vi "ABOUT SCREEN Unitest.vi"(8 "error in (no error)":errorcluster) -> (0 "error out":errorcluster)   [LabVIEW 2025]
panel:
  out "version":string="v1.AU.26"
  out "reference out":refnum<vi>
  in  "close":bool
  in  "Tab Selection":enum32{"About", "License", "Company"}(radio) caption="Radio Buttons - Customizable"
  out "Tab Control":T1(tab)
  out "Operating System":string="Windows 11 Pro"
  out "Version":string="1.AU.26"
  out "Workorder":string="2479"
  out "Runtime":string="LabVIEW 2025 (64-bit)"
  out "Instrument Serial":string="770073"
  out "Firmware Version":string="BCLV 3.6"
  # "v"
  # "© Copyright 2023 | Paltro Inc."
  # "All rights reserved."
  # "Version"
  # "Workorder"
  # "Runtime"
  # "Copyright"
  # "© 2023"
  # "Firmware Version"
  # "Operating System"
  # "Instrument Serial"
  # "Status"
  # "."
  # "Active"
  # "Licence Type"
  # "Single-seat commercial"
  # "Seats"
  # "1 of 1 in use"
  # "Expires"
  # "Perpetual"
  # "MANUFACTURER"
  # "Company"
  # "hello@palto.com"
  # "Mail"
  # "www.paltro.com"
  # "Website"
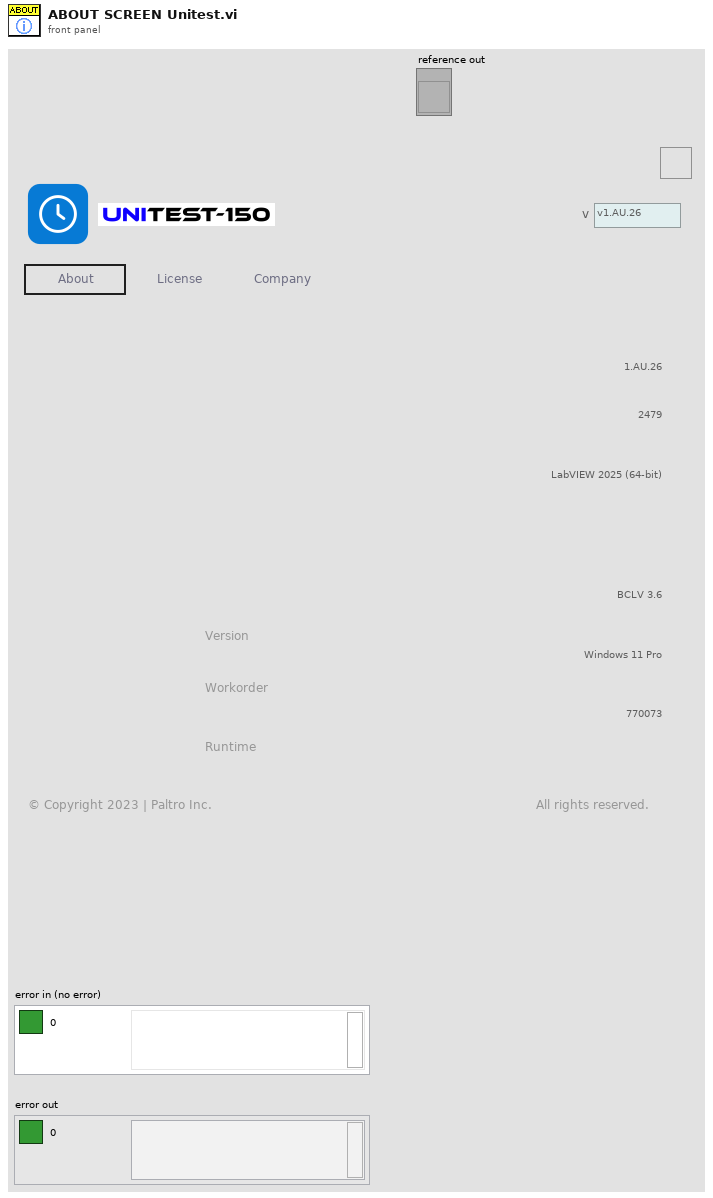
[diagram p1: front panel]
types:
  T1 = enum32{"About", "License", "Company", "System info"}
  T2 = enum32{"Invalid", "Standard", "Closed", "Hidden", "Minimized", "Maximized"}
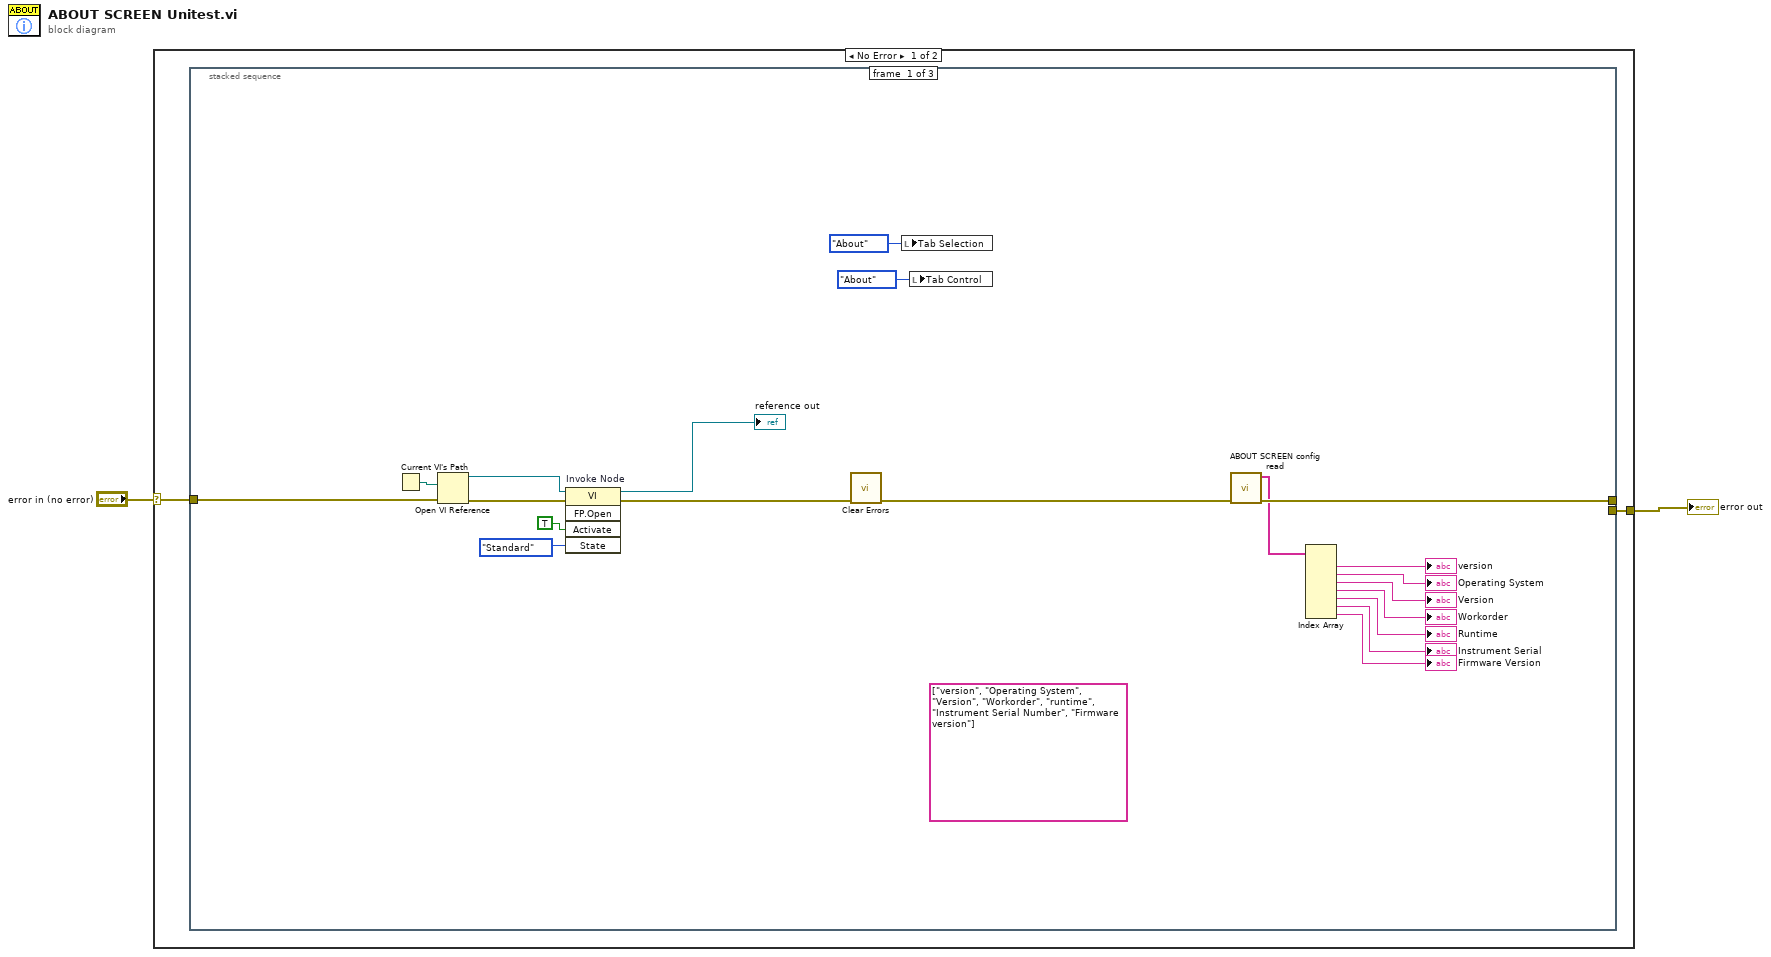
[diagram p0: block diagram]
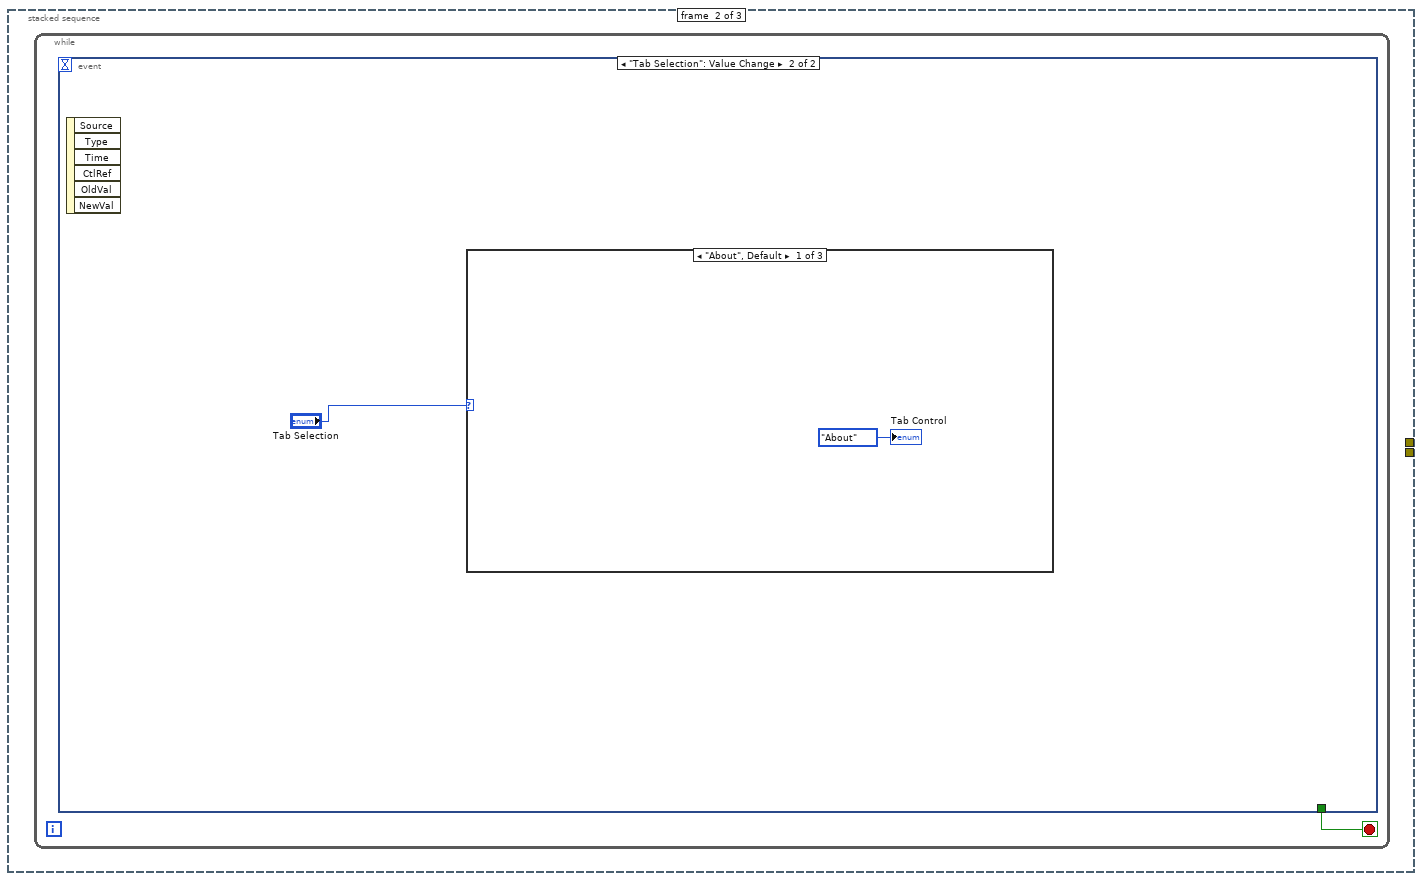
[diagram p2: hidden frame]
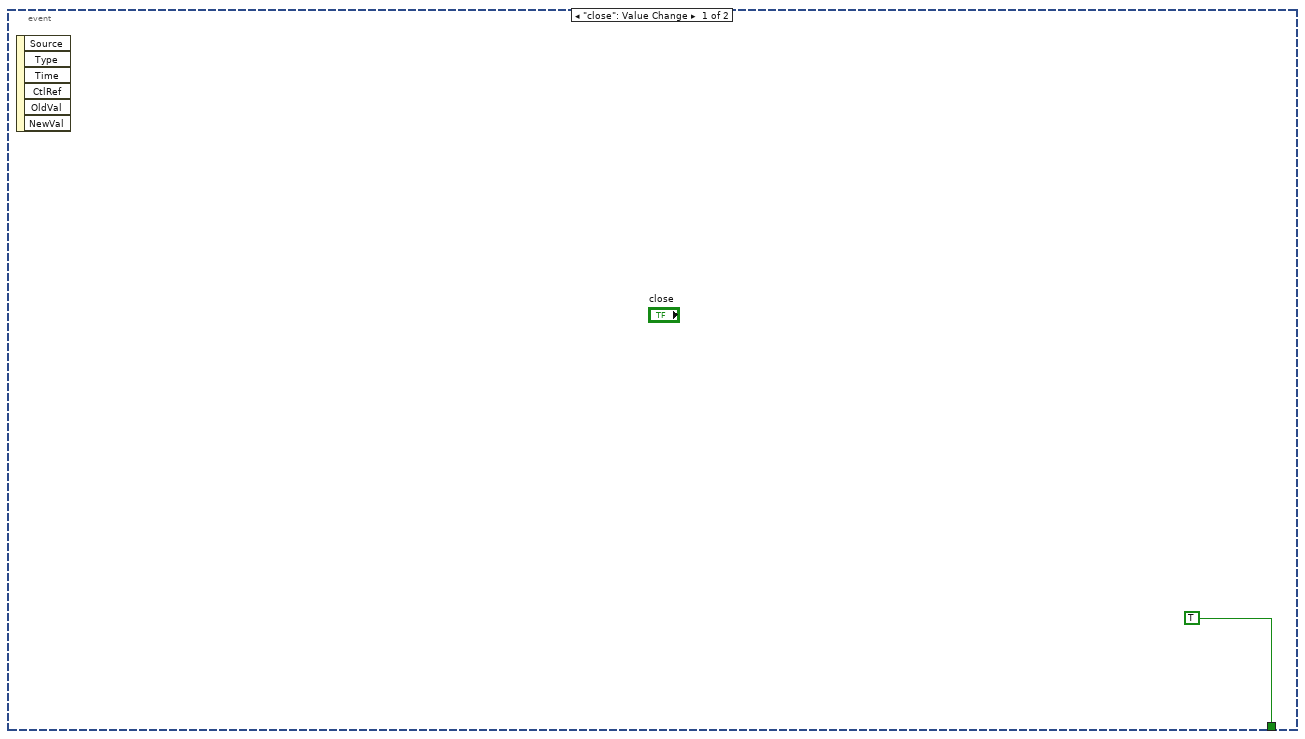
[diagram p3: hidden frame]
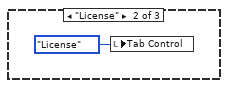
[diagram p4: hidden frame]
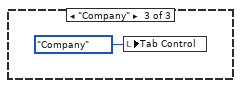
[diagram p5: hidden frame]
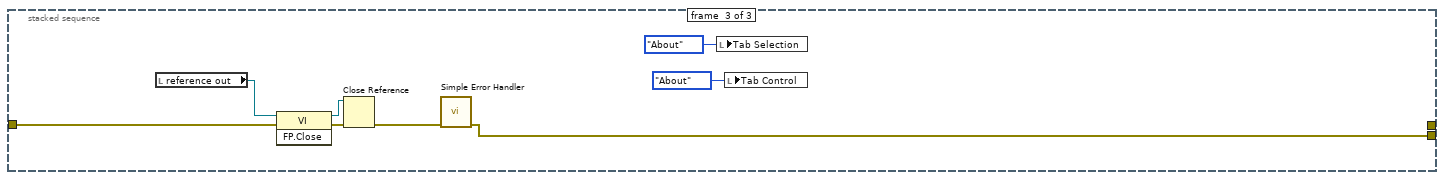
[diagram p6: hidden frame]
diagram:
  n1 = case shown="No Error" "error in (no error)" {
    selector: "error in (no error)" -> [w4 _]
    tunnel: [w3 _] -> w1
    frame No Error {
      n2 = stacked-sequence {
        tunnel: w4 -> [w19 _ w35]
        tunnel: [w13 _ _] -> _
        tunnel: [_ _ w33] -> w3
        frame #0 {
          (unwired) string[] ["version", "Operating System", "Version", "Workorder", "runtime", "Instrument Serial Number", "Firmware version"]
          n3 = Current VI's Path() -> (path=w24:path)
          n4 = Open VI Reference(vi path=w24, error in (no error)=w19) -> (vi reference=w20:refnum<vi>, error out=w21:errorcluster)  [unwired: 4 out]
          n5 = invoke on="Invoke Node" class="VI" method="FP.Open"(reference=w20, error in=w21, "Activate"=TRUE ("Activate?"), "State"=T2."Standard") -> (reference out=→"reference out":refnum<vi>, error out=w18:errorcluster)  [unwired: 1 in, 3 out]
          n6 = call <vilib>:"Clear Errors.vi"("error in (no error)"=w18) -> ("error out"=w14:errorcluster)  [unwired: 5 in, 1 out]
          n7 = local write "Tab Selection"(enum32{"About", "License", "Company"}."About" ("Tab Selection")) -> ()
          n8 = local write "Tab Control"(T1."About" ("Tab Control")) -> ()
          n9 = call "ABOUT SCREEN config read.vi"("error in (no error)"=w14) -> ("error out"=w13:errorcluster, "ABOUT SCREEN Parameters"=w12:string[])  [unwired: 9 in]
          n10 = Index Array(array=w12) -> (element #1=→"version":string, element #2=→"Operating System":string, element #3=→"Version":string, element #4=→"Workorder":string, element #5=→"Runtime":string, element #6=→"Instrument Serial":string, element #7=→"Firmware Version":string)  [unwired: 7 in]
        }
        frame #1 {
          n11 = while {
            stop <- w25 stop-if-true
            n12 = event shown="[1] \"Tab Selection\": Value Change" {
              selector: _ -> [_ _]
              dyn-events: _ -> [_ _]
              timeout: _ -> [_ _]
              tunnel: [TRUE _] -> w25
              event "close": Value Change {
                n13 = event-data() -> ()  [unwired: 1 in, 6 out]
              }
              event "Tab Selection": Value Change {
                n14 = event-data() -> ()  [unwired: 1 in, 6 out]
                n15 = case shown="\"About\", Default" "Tab Selection" {
                  frame "About", Default {
                    "Tab Control" <- T1."About" ("Tab Control")
                  }
                  frame "License" {
                    n16 = local write "Tab Control"(T1."License" ("Tab Control")) -> ()
                  }
                  frame "Company" {
                    n17 = local write "Tab Control"(T1."Company" ("Tab Control")) -> ()
                  }
                }
              }
            }
          }
        }
        frame #2 {
          n18 = local read "reference out"() -> (w34:refnum<vi>)
          n19 = invoke class="VI" method="FP.Close"(reference=w34, error in=w35) -> (reference out=w37:refnum<vi>, error out=w38:errorcluster)  [unwired: 1 in, 1 out]
          n20 = Close Reference(reference=w37, error in (no error)=w38) -> (error out=w36:errorcluster)
          n21 = call <vilib>:"Simple Error Handler.vi"("error in (no error)"=w36) -> ("error out"=w33:errorcluster)  [unwired: 1 in, 7 out]
          n22 = local write "Tab Selection"(enum32{"About", "License", "Company"}."About" ("Tab Selection")) -> ()
          n23 = local write "Tab Control"(T1."About" ("Tab Control")) -> ()
        }
      }
    }
    frame Error {
    }
  }
  "error out" <- w1
